vi "ex_GetHeaderFromChunk.vi"(8 "error in (no error)":errorcluster, 10 "chunk in":string, 11 "file ref in":T1={"file ref"=refnum, "file size (bytes:0)"=0, "read pointer (bytes:0)"=0, "chunk size (bytes:65000)"=65000}) -> (0 "error out":errorcluster, 1 "header":string, 2 "chunk remainder":string, 3 "file ref out":T1={"file ref"=refnum, "file size (bytes:0)"=0, "read pointer (bytes:0)"=0, "chunk size (bytes:65000)"=65000}, 4 "end of file?":bool, 5 "special blocks":string[](array[string]), 6 "no header?":bool)   [LabVIEW 2020]
uses:
  express shared/ExFile.llb/ex_FileReference.ctl
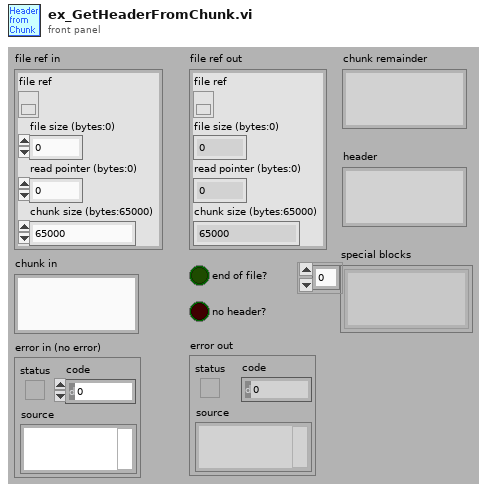
[diagram p1: front panel]
types:
  T1 = typedef "ex_FileReference.ctl" = cluster{"file ref":refnum<file>, "file size (bytes:0)":i32, "read pointer (bytes:0)":i32, "chunk size (bytes:65000)":i32}
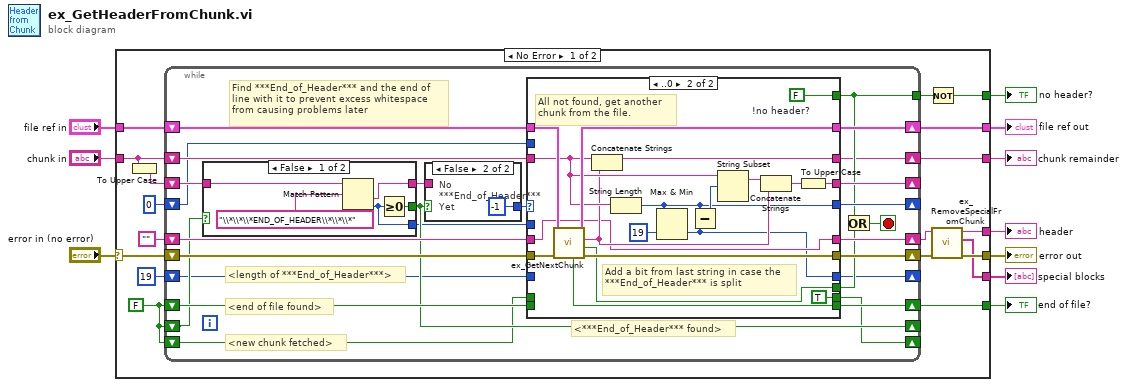
[diagram p0: block diagram]
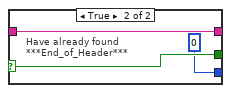
[diagram p2: hidden frame]
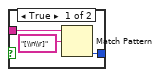
[diagram p3: hidden frame]
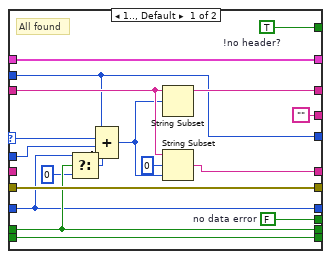
[diagram p4: hidden frame]
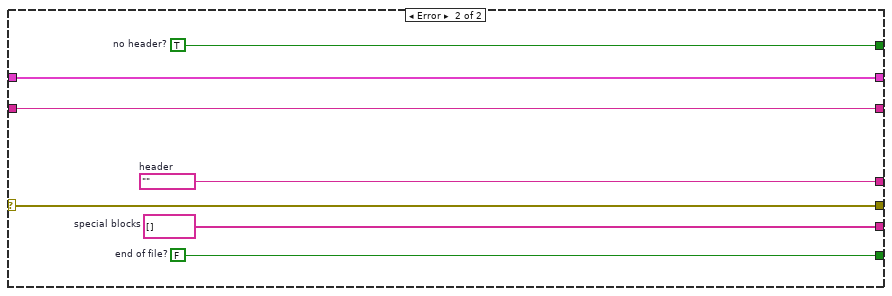
[diagram p5: hidden frame]
diagram:
  n1 = case shown="No Error" "error in (no error)" {
    selector: "error in (no error)" -> [w27 w110]
    tunnel: "chunk in" -> [w14 w109]
    tunnel: [w13 w109] -> w9
    tunnel: [w18 w110] -> w1
    tunnel: [w19 w106] -> w8
    tunnel: [w17 w105] -> w7
    tunnel: [w16 w107] -> w6
    tunnel: [w25 w108] -> w3
    tunnel: "file ref in" -> [w26 w108]
    tunnel: [w15 w104] -> w2
    frame No Error {
      w12 = FALSE
      n2 = To Upper Case(1:w14) -> (0:w23:string)
      n3 = while {
        tunnel: [w42] -> w28
        shift-right: [w53] -> w20
        shift-left: w27 -> [w54]
        shift-right: [w51] -> w25
        shift-left: w26 -> [w52]
        shift-right: [w50] -> w21
        shift-left: "" -> [w49]
        shift-right: [w46] -> _
        shift-left: w23 -> [w48]
        shift-right: [w47] -> _
        shift-left: 0 ("offset (0)") -> [w31]
        shift-right: [w45] -> w15
        shift-left: w12 -> [w44]
        shift-right: [w39] -> w13
        shift-left: w14 -> [w40]
        shift-right: [w35] -> _
        shift-left: w12 -> [w36]
        shift-right: [w33] -> _
        shift-left: w12 -> [w32]
        shift-right: [w29] -> _
        shift-left: 19 ("length of ***End_of_Header***") -> [w30]
        stop <- w41 stop-if-true
        # "<length of ***End_of_Header***>"
        # "<***End_of_Header*** found>"
        # "<end of file found>"
        # "<new chunk fetched>"
        # "Find ***End_of_Header*** and the end of\nline with it to prevent excess whitespace\nfrom causing problems later"
        n4 = case shown="False" w36 {
          selector: w36 -> [_ w61]
          tunnel: w48 -> [w58 w62]
          tunnel: [w57 w62] -> w38
          tunnel: [w55 w61] -> w35
          tunnel: [w56 0 ("offset past match")] -> w34
          frame False {
            n5 = Match Pattern(string=w58, regular expression="\\*\\*\\*END_OF_HEADER\\*\\*\\*") -> (after substring=w57:string, offset past match=w56:i32)  [unwired: 3 out]
            n6 = Greater Or Equal To 0?(x=w56) -> (x >= 0?=w55:bool)
          }
          frame True {
            # "Have already found\n***End_of_Header***"
          }
        }
        n7 = case shown="False" w35 {
          tunnel: w38 -> [w64 _]
          tunnel: [w63 -1 ("offset past match")] -> w37
          frame True {
            n8 = Match Pattern(string=w64, regular expression="[\\n\\r]") -> (offset past match=w63:i32)  [unwired: 4 out]
          }
          frame False {
            # "No\n***End_of_Header***\nYet"
          }
        }
        n9 = case shown="..0" w37 {
          selector: w37 -> [w74 _]
          tunnel: w40 -> [w83 w95]
          tunnel: [w84 w98] -> w39
          tunnel: w54 -> [w79 w101]
          tunnel: [w79 w97] -> w53
          tunnel: w30 -> [w67 _]
          tunnel: [w78 w88] -> w50
          tunnel: [w82 w103] -> w42
          tunnel: w52 -> [w80 w102]
          tunnel: [w80 w100] -> w51
          tunnel: w49 -> [_ w88]
          tunnel: [w73 w87] -> w47
          tunnel: ["" w99] -> w46
          tunnel: w31 -> [w73 _]
          tunnel: [w77 w96] -> w45
          tunnel: [w76 w89] -> w43
          tunnel: w44 -> [w77 _]
          tunnel: w34 -> [w72 _]
          tunnel: [w69 TRUE] -> w33
          tunnel: w32 -> [w69 _]
          tunnel: [w67 w85] -> w29
          frame 1.., Default {
            w76 = FALSE  # no data error
            w82 = TRUE  # !no header?
            # "All found"
            n10 = Select(t=w67, s=w69, f=0) -> (s? t:f=w70:i32)
            n11 = Compound Arithmetic op=ADD(w73, w74, w72, invert w70) -> (w71:i32)
            n12 = String Subset(string=w83, offset (0)=w71) -> (substring=w84:string)  [unwired: 1 out]
            n13 = String Subset(string=w83, offset (0)=0, length (rest)=w71) -> (substring=w78:string)
          }
          frame ..0 {
            w103 = FALSE  # !no header?
            # "All not found, get another\nchunk from the file."
            # "Add a bit from last string in case the\n***End_of_Header*** is split"
            n14 = call "ex_GetNextChunk.vi"("error in (no error)"=w101, "file refs"=w102) -> ("error out"=w97:errorcluster, "no data error"=w89:bool, "chunk"=w92:string, "dup file refs"=w100:T1, "end-of-file?"=w96:bool)  [unwired: 5 out]
            n15 = Concatenate Strings(w95, w92) -> (w98:string)
            n16 = String Length(string=w95) -> (length=w87:i32)
            n17 = Max & Min(x=w87, y=19) -> (min(x,y)=w85:i32)  [unwired: 1 out]
            n18 = Subtract(x=w87, y=w85) -> (x-y=w91:i32)
            n19 = String Subset(string=w95, offset (0)=w91) -> (substring=w93:string)  [unwired: 1 out]
            n20 = Concatenate Strings(w93, w92) -> (w94:string)
            n21 = To Upper Case(1:w94) -> (0:w99:string)
          }
        }
        n22 = Or(x=w42, y=w43) -> (x .or. y?=w41:bool)
      }
      n23 = Not(x=w28) -> (.not. x?=w16:bool)
      n24 = call "ex_RemoveSpecialFromChunk.vi"("error in (no error)"=w20, "chunk in"=w21) -> ("error out"=w18:errorcluster, "special blocks"=w17:string[], "chunk remainder"=w19:string)  [unwired: 7 out]
    }
    frame Error {
      w105 = string[] []  # special blocks
      w104 = FALSE  # end of file?
      w106 = ""  # header
      w107 = TRUE  # no header?
    }
  }
  "chunk remainder" <- w9
  "header" <- w8
  "special blocks" <- w7
  "no header?" <- w6
  "error out" <- w1
  "file ref out" <- w3
  "end of file?" <- w2
